vi "Prune.vi"(8 "error in (no error)":errorcluster, 10 "Master Device in":refnum<class "Master Device.lvclass">, 11 "Arduino in":refnum<class "Arduino.lvclass">) -> (0 "error out":errorcluster, 2 "Master Device out":refnum<class "Master Device.lvclass">, 3 "Arduino out":refnum<class "Arduino.lvclass">)   [LabVIEW 2013, in "Arduino.lvclass"]
doc: "Prune.vi is the first of two subVIs called in FinalizeHWI. Triggered slave devices need to:\n (1) Re-check triggering from Master Device's \"Slave Info\" to see what ramps are required to be programmed\n (2) Prune those lines from the \"prepared\" image (in reversed order just like triggering and the Ramp List) that will not be triggered.\n\nThe next subVI called is BuildHWI where you will actually flatten the \"prepared\" image and put it in normal time order."
uses:
  Arduino.lvclass
  Device/Device.lvclass
  Master Device/Master Device.lvclass
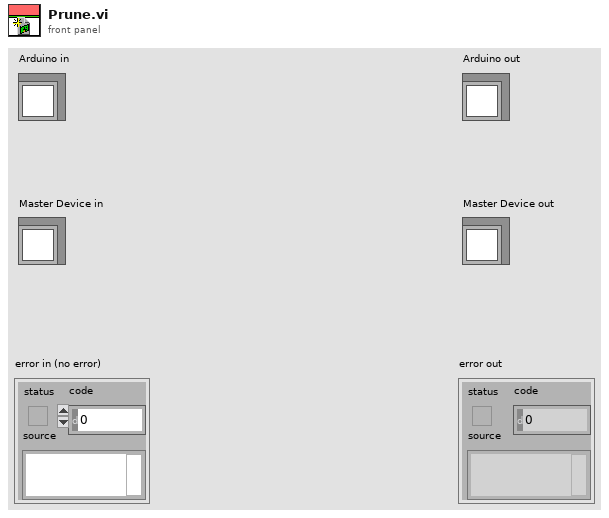
[diagram p1: front panel]
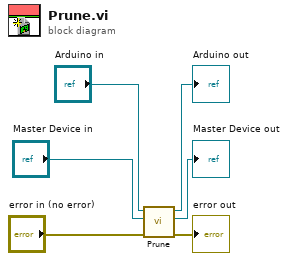
[diagram p0: block diagram]
diagram:
  n1 = call-parent "Prune.vi"("error in (no error)"="error in (no error)", "Master Device in"="Master Device in", "Device in"="Arduino in") -> ("error out"=→"error out":errorcluster, "Master Device out"=→"Master Device out":refnum<class "Master Device.lvclass">, "Device out"=→"Arduino out":refnum<class "Arduino.lvclass">)  [unwired: 6 in]
